vi "直通基准测试.vi"   [LabVIEW 2011]
uses:
  network/network.lvclass
types:
  T1 = typedef "直通基准state.ctl" = enum16{"开始消息", "切换开关"}
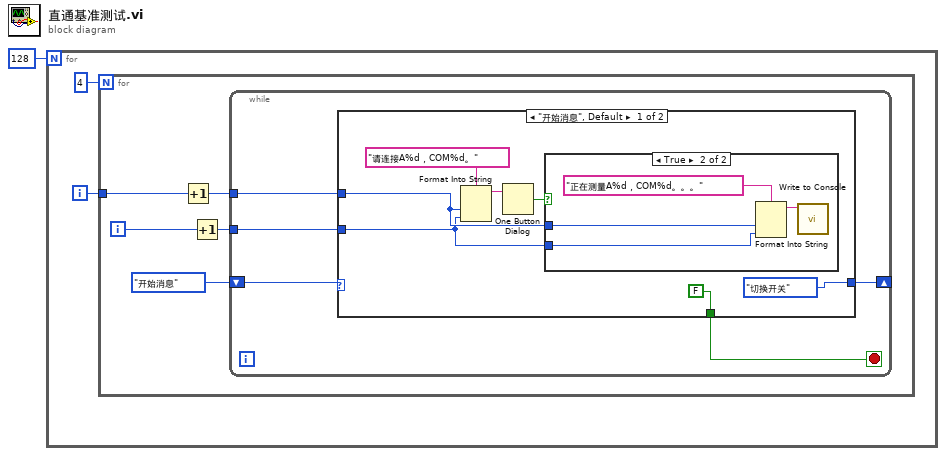
[diagram p0: block diagram]
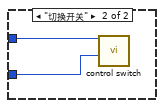
[diagram p3: hidden frame]
diagram:
  n1 = for {
    N: 128 -> [_]
    i -> [w2]
    n2 = for {
      N: 4 -> [_]
      tunnel: w2 -> [w8]
      i -> [w7]
      n3 = Increment(x=w8) -> (x+1=w6:i32)
      n4 = Increment(x=w7) -> (x+1=w5:i32)
      n5 = while {
        tunnel: w6 -> [w13]
        tunnel: w5 -> [w12]
        shift-right: [w10] -> _
        shift-left: 直通基准state."开始消息" ("直通基准State") -> [w11]
        stop <- w9 stop-if-true
        n6 = case shown="\"开始消息\", Default" w11 {
          tunnel: w13 -> [w20 w26]
          tunnel: w12 -> [w19 w25]
          tunnel: [直通基准state."切换开关" ("直通基准State") _] -> w10
          tunnel: [FALSE _] -> w9
          frame "开始消息", Default {
            n7 = Format Into String(format string="请连接A%d，COM%d。", w20, w19) -> (resulting string=w17:string)  [unwired: 2 in, 1 out]
            n8 = One Button Dialog(message=w17) -> (true=w16:bool)  [unwired: 1 in]
            n9 = case shown="True" w16 {
              tunnel: w20 -> [_ w23]
              tunnel: w19 -> [_ w22]
              frame False {
              }
              frame True {
                n10 = Format Into String(format string="正在测量A%d，COM%d。。。", w23, w22) -> (resulting string=w21:string)  [unwired: 2 in, 1 out]
                n11 = call "Write to Console.vi"("Input"=w21) -> ()  [unwired: 10 in, 1 out]
              }
            }
          }
          frame "切换开关" {
            n12 = call "control switch.vi"("COM"=w25, "A"=w26) -> ()  [unwired: 9 in, 1 out]
          }
        }
      }
    }
  }
